vi "Get JSON Example.vi"(6 "type":enum16{"request", "response"}(ring), 8 "error in (no error)":errorcluster, 9 "params":variant, 10 "method":string) -> (0 "error out":errorcluster, 2 "<JSON>":string)   [LabVIEW 2019, in "Help.lvclass"]
uses:
  Help.lvclass
  <userlib>/LevyLab/JSON-RPC/JSON-RPC.lvlib
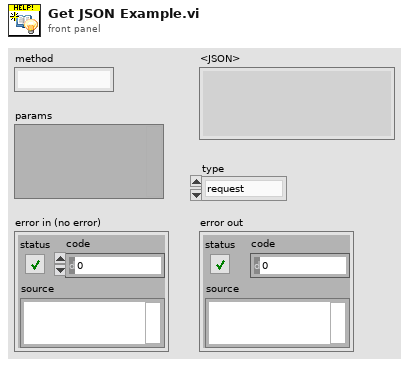
[diagram p1: front panel]
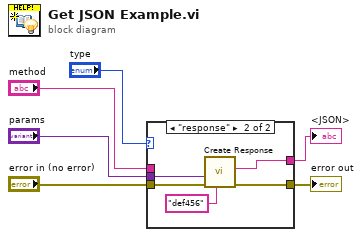
[diagram p0: block diagram]
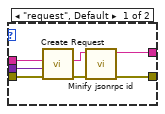
[diagram p2: hidden frame]
diagram:
  n1 = case shown="\"response\"" "type" {
    tunnel: [w13 w15] -> w6
    tunnel: "error in (no error)" -> [w12 w18]
    tunnel: "method" -> [w10 _]
    tunnel: "params" -> [w9 w17]
    tunnel: [w8 w14] -> w2
    frame "request", Default {
      n2 = call <userlib>:"Create Request.vi"("error in (no error)"=w12, "params"=w9, "method"=w10) -> ("error out"=w11:errorcluster, "<JSON> Requests"=w7:string)  [unwired: 6 in, 1 out]
      n3 = call "Minify jsonrpc id.vi"("error in (no error)"=w11, "<JSON> Requests"=w7) -> ("error out"=w13:errorcluster, "<JSON>"=w8:string)  [unwired: 8 in]
    }
    frame "response" {
      n4 = call <userlib>:"Create Response.vi"("id"="def456", "error in (no error)"=w18, "result"=w17) -> ("error out"=w15:errorcluster, "<JSON> Response"=w14:string)  [unwired: 7 in]
    }
  }
  "error out" <- w6
  "<JSON>" <- w2
